vi "Robot Init (SubVI).vi"() -> (0 "Fehler (Ausgang)":errorcluster, 3 "robot session*":string)   [LabVIEW 2013]
uses:
  <vilib>/ImagingLab/Kawasaki Robotics Library/typedefs/KwRL-Eth_parameters.ctl
  <vilib>/ImagingLab/Kawasaki Robotics Library/typedefs/KwRL-coordinate_system.ctl
  <vilib>/ImagingLab/Kawasaki Robotics Library/typedefs/KwRL-cartesian.ctl
  <vilib>/ImagingLab/Kawasaki Robotics Library/typedefs/KwRL-on_off.ctl
  <vilib>/ImagingLab/Kawasaki Robotics Library/typedefs/KwRL-joint_displacement.ctl
  <vilib>/ImagingLab/Kawasaki Robotics Library/sub/poly/kwrl-motion-parameters_set_speed(monitor).vi
  <vilib>/ImagingLab/Kawasaki Robotics Library/KawasakiRoboticsLibrary.lvlib
panel:
  in  "ethernet connection settings":T1={"IP1 port"=49152, "IP2 port"=49153, "TELNET port"=23, "robot IP address"="10.10.14.198"}
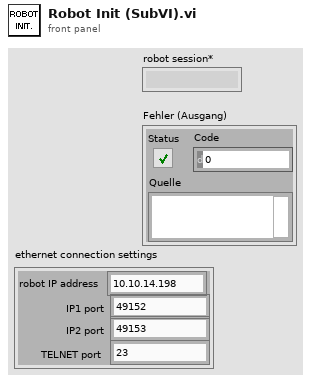
[diagram p1: front panel]
types:
  T1 = typedef "KawasakiRoboticsLibrary.lvlib/KwRL-Eth_parameters.ctl" = cluster{"IP1 port":u16, "IP2 port":u16, "TELNET port":u16, "robot IP address":string}
  T2 = typedef "KawasakiRoboticsLibrary.lvlib/KwRL-joint_displacement.ctl" = cluster{"JT1":dbl, "JT2":dbl, "JT3":dbl, "JT4":dbl, "JT5":dbl, "JT6":dbl, "JT7":dbl}
  T3 = typedef "KawasakiRoboticsLibrary.lvlib/KwRL-on_off.ctl" = dbl
  T4 = typedef "KawasakiRoboticsLibrary.lvlib/KwRL-cartesian.ctl" = cluster{"X":dbl, "Y":dbl, "Z":dbl, "O":dbl, "A":dbl, "T":dbl, "S":dbl}
  T5 = typedef "KawasakiRoboticsLibrary.lvlib/KwRL-coordinate_system.ctl" = enum16{"BASE", "TOOL"}
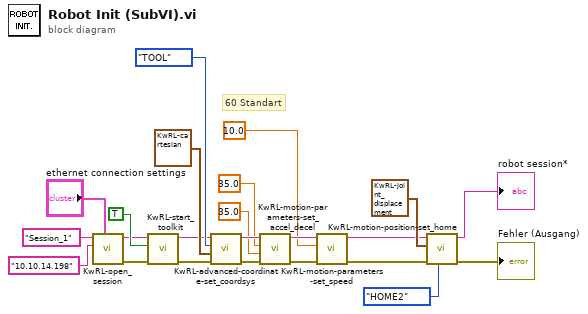
[diagram p0: block diagram]
diagram:
  # "60 Standart"
  n1 = call <vilib>:"KwRL-open_session.vi"("ethernet connection settings"="ethernet connection settings", "robot IP address"="10.10.14.198", "robot session"="Session_1") -> ("error out"=w13:errorcluster, "robot session*"=w14:string)  [unwired: 6 in, 1 out]
  n2 = call <vilib>:"KwRL-start_toolkit.vi"("error in"=w13, "full start"=TRUE, "robot session"=w14) -> ("error out"=w18:errorcluster, "robot session*"=w20:string)  [unwired: 6 in, 1 out]
  n3 = call <vilib>:"KwRL-advanced-coordinate-set_coordsys.vi"("error in"=w18, "position"=T4 {"X"=-60.0, "Y"=0.0, "Z"=59.0, "O"=0.0, "A"=180.0, "T"=0.0, "S"=0.0} ("position 3"), "coordinate system"=KwRL-coordinate_system."TOOL", "robot session"=w20) -> ("error out"=w19:errorcluster, "robot session*"=w21:string)  [unwired: 6 in]
  n4 = call <vilib>:"KwRL-motion-parameters-set_accel_decel.vi"("error in"=w19, "deceleration"=T3 35.0, "acceleration"=T3 35.0, "robot session"=w21) -> ("error out"=w10:errorcluster, "robot session*"=w9:string)  [unwired: 6 in]
  n5 = call-poly <vilib>:"KwRL-motion-parameters-set_speed.vi"("error in"=w10, "speed (%)"=T3 10.0, "robot session"=w9) -> ("error out"=w6:errorcluster, "robot session*"=w2:string)  [unwired: 7 in]
  n6 = call <vilib>:"KwRL-motion-position-set_home.vi"("home position"=enum16{"HOME", "HOME2"}."HOME2", "error in"=w6, "joint displacement"=T2 {"JT1"=0.0, "JT2"=-30.0, "JT3"=-120.0, "JT4"=0.0, "JT5"=-90.0, "JT6"=90.0, "JT7"=0.0} ("joint displacement 2"), "robot session"=w2) -> ("error out"=→"Fehler (Ausgang)":errorcluster, "robot session*"=→"robot session*":string)  [unwired: 6 in]
